vi "Set Task Base.vi"(8 "error in (no error)":errorcluster, 10 "HAL GOOP4.lvlib:Task Base.lvclass":refnum<class "Task Base.lvclass">, 11 "Task Actor in":refnum<class "Task Actor.lvclass">) -> (0 "error out":errorcluster, 3 "Task Actor out":refnum<class "Task Actor.lvclass">)   [LabVIEW 2023, in "Task Actor.lvlib" / "Task Actor.lvclass"]
uses:
  Task Actor.lvclass
  Task Base/Task Base.lvclass
  Task Actor.lvclass/Task Actor.ctl
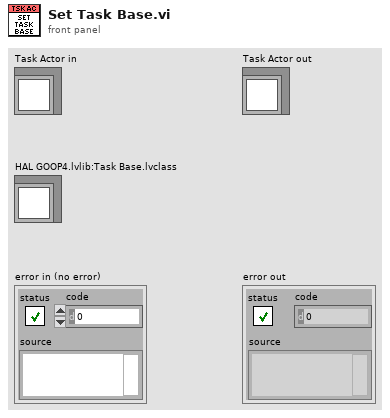
[diagram p1: front panel]
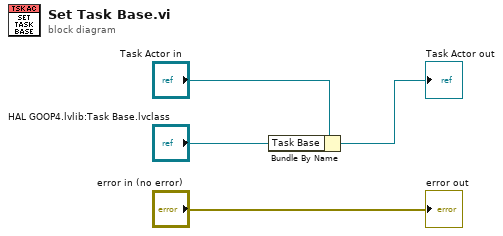
[diagram p0: block diagram]
diagram:
  n1 = Bundle By Name(cluster="Task Actor in", "Task Base"="HAL GOOP4.lvlib:Task Base.lvclass") -> (→"Task Actor out":refnum<class "Task Actor.lvclass">)
  "error out" <- "error in (no error)"
